vi "string2cmds Rigid Joystick.vi"(7 "numCmds":i32=11, 11 "input string":string) -> (3 "output cmds":dbl[](array[numeric]))   [LabVIEW 2016]
panel:
  # ">>>"
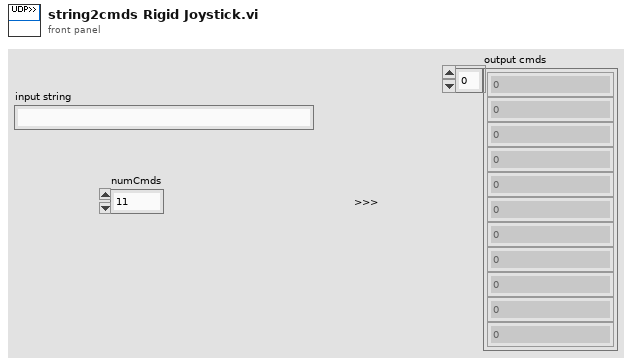
[diagram p1: front panel]
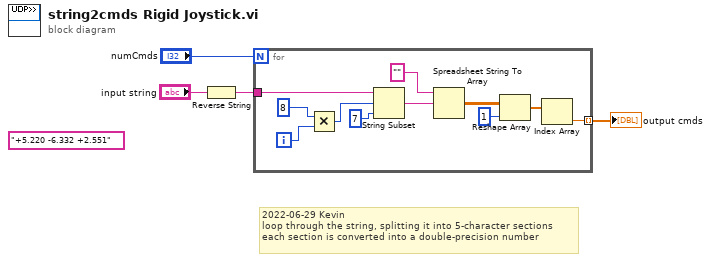
[diagram p0: block diagram]
diagram:
  (unwired) "+5.220 -6.332 +2.551" ("input string 2")
  # "2022-06-29 Kevin\nloop through the string, splitting it into 5-character sections\neach section is converted into a double-precision number"
  n1 = Reverse String(1:"input string") -> (0:w1:string)
  n2 = for {
    N: "numCmds" -> [_]
    tunnel: w1 -> [w12]
    tunnel: [w6] -> w3 mode=indexing
    i -> [w5]
    n3 = Multiply(x=8, y=w5) -> (x*y=w13:i32)
    n4 = String Subset(string=w12, offset (0)=w13, length (rest)=7 ("offset (0)")) -> (substring=w11:string)
    n5 = Spreadsheet String To Array(format string="", spreadsheet string=w11) -> (array=w8:dbl[][])  [unwired: 2 in]
    n6 = Reshape Array(w8, 1 ("dimension size")) -> (w7:dbl[])
    n7 = Index Array(array=w7) -> (element=w6:dbl)  [unwired: 1 in]
  }
  "output cmds" <- w3
